vi "Read Digital Port.vi"(8 "error in (no error)":errorcluster, 11 "DIO in":refnum<class "DIO.lvclass">) -> (0 "error out":errorcluster, 2 "Relay Mode":bool[](array[boolean]), 3 "DIO out":refnum<class "DIO.lvclass">)   [LabVIEW 2019, in "Hardware Abstration.lvlib" / "DIO.lvclass"]
uses:
  DIO.lvclass
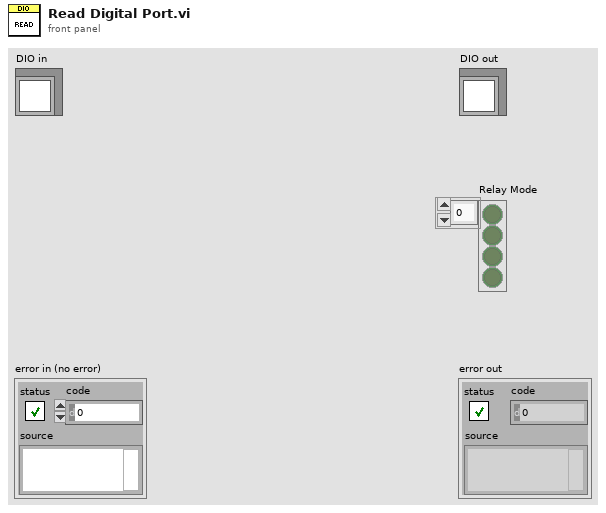
[diagram p1: front panel]
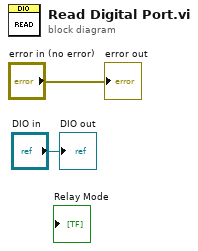
[diagram p0: block diagram]
diagram:
  "error out" <- "error in (no error)"
  "DIO out" <- "DIO in"
